vi "Initialize Front Panel.vi"(8 "error in (no error)":errorcluster, 11 "TwoPaneViewManager in":refnum<class "TwoPaneViewManager.lvclass">) -> (0 "error out":errorcluster, 3 "TwoPaneViewManager out":refnum<class "TwoPaneViewManager.lvclass">)   [LabVIEW 2020, in "MVAExamples.lvlib" / "TwoPaneViewManager.lvclass"]
doc: "<License>\nCopyright © 2017 Composed Systems, LLC | All rights reserved\nwww.composed.io\n\nAuthor: Ethan Stern <ethan.stern@composed.io>\n\nThis software is provided \"AS IS\" WITHOUT WARRANTIES, either express or implied, AND IS FOR EDUCATIONAL PURPOSES ONLY.\n</License>"
uses:
  TwoPaneViewManager.lvclass
  modules/mva-viewable/Source/IViewManager/IViewManager/IViewManager.lvclass/IViewManager.ctl
  TwoPaneViewManager.lvclass/TwoPaneViewManager.ctl
  modules/mva-viewable/Source/IViewable/IViewable Messages/Insert Front Panel Msg/Insert Front Panel Msg.lvclass/Insert Front Panel Msg.ctl
  <vilib>/ActorFramework/Message Enqueuer/Message Enqueuer.lvclass/Message Enqueuer.ctl
  <vilib>/ActorFramework/Message Enqueuer/Enqueue.vi
  modules/mva-viewable/Source/IViewable/IViewable Messages/Insert Front Panel Msg/Insert Front Panel Msg.lvclass
  C:/Program Files/National Instruments/LabVIEW 2020/vi.lib/ActorFramework/Message/Message.lvclass
  <vilib>/ActorFramework/Message Priority Queue/Priority Enqueue.vi
  modules/mva-viewable/Source/IViewManager/IViewManager/IViewManager.lvclass
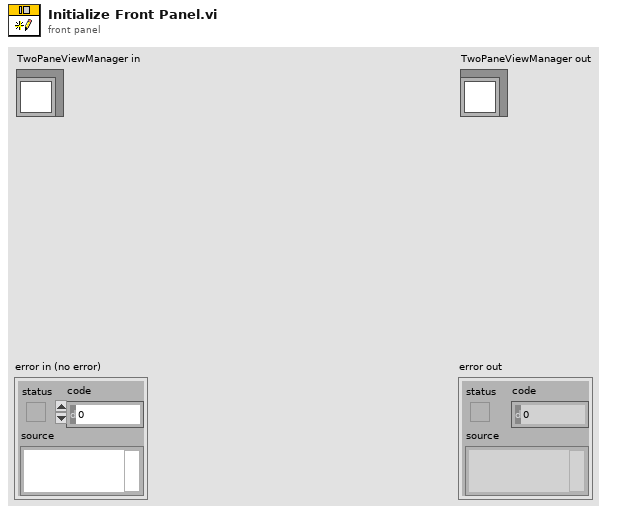
[diagram p1: front panel]
types:
  T1 = typedef "IViewable.lvlib/ProtectedSubpanel.lvclass/Protected Subpanel Reference.ctl" = refnum<data-value>
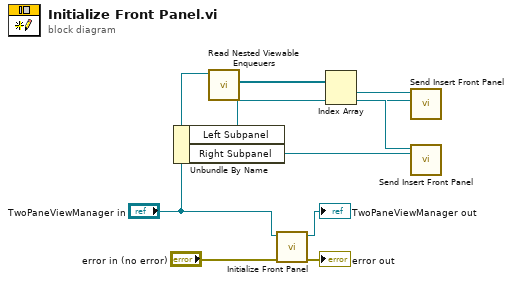
[diagram p0: block diagram]
diagram:
  n1 = Unbundle By Name("TwoPaneViewManager in") -> ("Left Subpanel"=w2:T1, "Right Subpanel"=w1:T1)
  n2 = call "Read Nested Viewable Enqueuers.vi"("IViewManager in"="TwoPaneViewManager in") -> ("Nested Viewable Enqueuers"=w5:refnum<class "Message Enqueuer.lvclass">[])  [unwired: 9 in, 1 out]
  n3 = call-parent "Initialize Front Panel.vi"("error in (no error)"="error in (no error)", "IViewable in"="TwoPaneViewManager in") -> ("error out"=→"error out":errorcluster, "IViewable out"=→"TwoPaneViewManager out":refnum<class "TwoPaneViewManager.lvclass">)  [unwired: 8 in]
  n4 = Index Array(array=w5) -> (element #1=w4:refnum<class "Message Enqueuer.lvclass">, element #2=w3:refnum<class "Message Enqueuer.lvclass">)  [unwired: 2 in]
  n5 = call "Send Insert Front Panel.vi"("Protected Subpanel"=w2, "Message Enqueuer"=w4) -> ()  [unwired: 8 in, 2 out]
  n6 = call "Send Insert Front Panel.vi"("Protected Subpanel"=w1, "Message Enqueuer"=w3) -> ()  [unwired: 8 in, 2 out]
